vi "idk.vi"() -> ()   [LabVIEW 2019]
uses:
  <vilib>/Analysis/NI_AALPro.lvlib
  <vilib>/ptbypt/NI_PtbyPt.lvlib
panel:
  out "Waveform Chart 3":dbl[](graph)
  out "Waveform Chart 2":dbl[](graph)
  out "Waveform Chart":dbl[](graph)
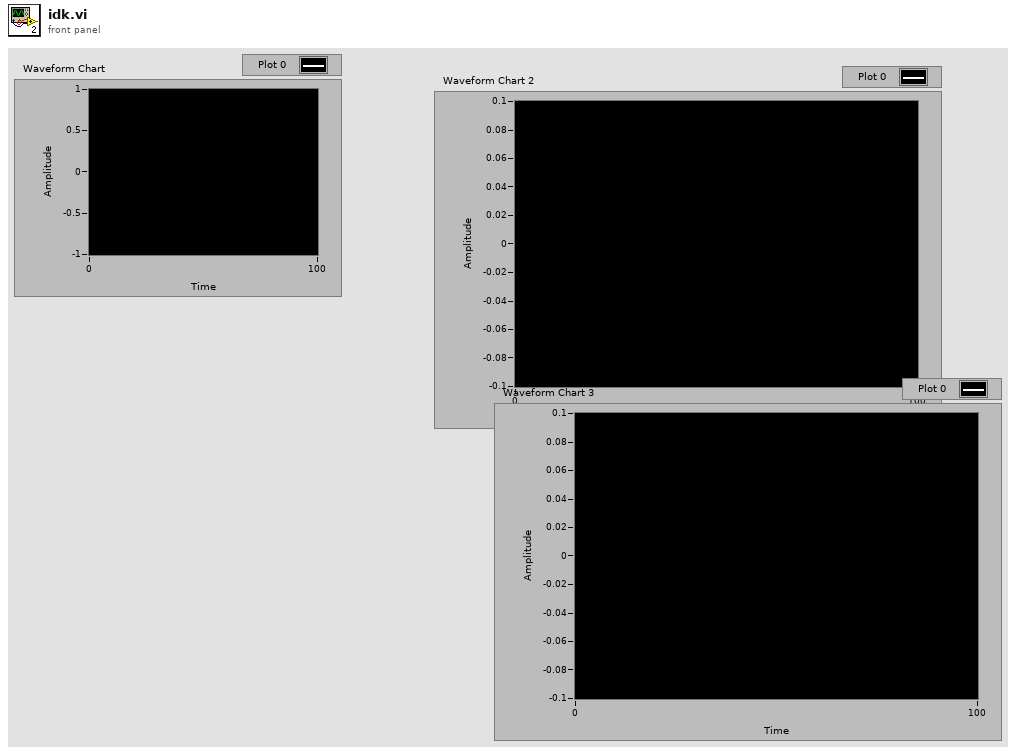
[diagram p1: front panel]
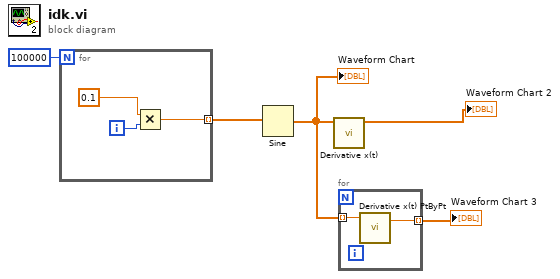
[diagram p0: block diagram]
diagram:
  n1 = for {
    N: 100000 -> [_]
    tunnel: [w6] -> w4 mode=indexing
    i -> [w8]
    n2 = Multiply(x=0.1, y=w8) -> (x*y=w6:dbl)
  }
  n3 = Sine(x=w4) -> (sin(x)=w2:dbl[])
  "Waveform Chart" <- w2
  n4 = call <vilib>:"Derivative x(t).vi"("X"=w2) -> ("dX/dt"=→"Waveform Chart 2":dbl[])  [unwired: 9 in, 1 out]
  n5 = for {
    tunnel: w2 -> [w10] mode=indexing
    tunnel: [w9] -> w1 mode=indexing
    n6 = call <vilib>:"Derivative x(t) PtByPt.vi"("x"=w10) -> ("dx/dt"=w9:dbl)  [unwired: 3 in, 1 out]
  }
  "Waveform Chart 3" <- w1
